vi "06T_Open_connection.vi"(10 "Period, ms":dbl=50.0 min=10.0 max=10000.0, 11 "COM port":refnum<visa-resource-name>) -> (3 "VISA":refnum<visa-resource-name>)   [LabVIEW 2013]
uses:
  <vilib>/Instr/_visa.llb/VISA Configure Serial Port (Instr).vi
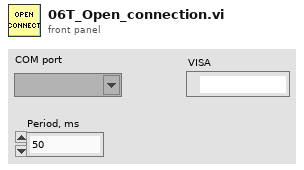
[diagram p1: front panel]
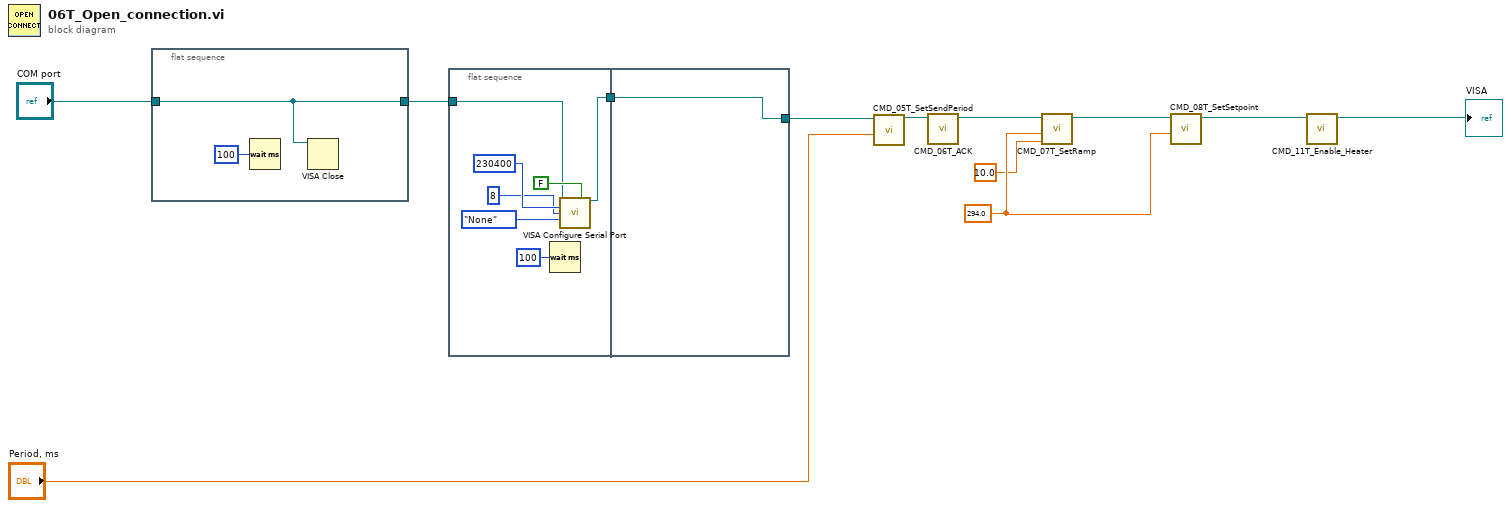
[diagram p0: block diagram]
diagram:
  w2 = 294.0 ("Setpoint, K")
  n1 = flat-sequence {
    tunnel: [w13] -> w11
    tunnel: "COM port" -> [w13]
    frame #0 {
      n2 = Wait (ms)(milliseconds to wait=u32 100) -> ()  [unwired: 1 out]
      n3 = VISA Close(VISA resource name=w13) -> ()  [unwired: 1 in, 1 out]
    }
  }
  n4 = flat-sequence {
    tunnel: w11 -> [w17]
    tunnel: [w16] -> w12
    tunnel: [w22] -> w9
    tunnel: w12 -> [w22]
    frame #0 {
      n5 = Wait (ms)(milliseconds to wait=u32 100) -> ()  [unwired: 1 out]
      n6 = call-poly "VISA Configure Serial Port"("VISA resource name"=w17, "Enable Termination\nChar (T)"=FALSE ("Enable Termination\nChar (T)"), "baud rate (9600)"=u32 230400, "data bits (8)"=u16 8, "parity (0:none)"=enum16{"None", "Odd", "Even", "Mark", "Space"}."None") -> ("VISA resource name out"=w16:refnum<visa-resource-name>)  [unwired: 9 in, 1 out]
    }
    frame #1 {
    }
  }
  n7 = call "CMD_05T_SetSendPeriod.vi"("Period, ms"="Period, ms", "VISA resource name"=w9) -> ("VISA resource name out"=w10:refnum<visa-resource-name>)  [unwired: 9 in]
  n8 = call "CMD_06T_ACK.vi"("VISA resource name"=w10) -> ("VISA resource name out"=w4:refnum<visa-resource-name>)  [unwired: 10 in]
  n9 = call "CMD_07T_SetRamp.vi"("Ramp speed, K/min"=10.0, "Target, K"=w2, "VISA resource name"=w4) -> ("VISA resource name out"=w3:refnum<visa-resource-name>)  [unwired: 8 in]
  n10 = call "CMD_08T_SetSetpoint.vi"("Setpoint, K"=w2, "VISA resource name"=w3) -> ("VISA resource name out"=w8:refnum<visa-resource-name>)  [unwired: 9 in]
  n11 = call "CMD_11T_Enable_Heater.vi"("VISA resource name"=w8) -> ("VISA resource name out"=→"VISA":refnum<visa-resource-name>)  [unwired: 10 in]
